vi "PmacProgParse.vi"(1 "Program Buffer String":string) -> (0 "Program VI State Cluster":T1={"Program Loaded"=FALSE, "Program Number i32"=1, "Coord Number i32"=1} {"Coord Number i32" min=1 max=8; "Program Number i32" min=1})   [LabVIEW 2020]
doc: "Parse Program Buffer to Program Number and Coord Number to run the program in. Provide the information in Program VI State Cluster. The program load state is not determined by this operation."
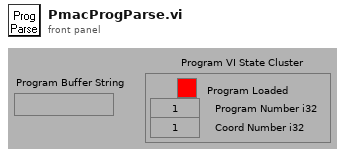
[diagram p1: front panel]
types:
  T1 = cluster{"Program Loaded":bool, "Program Number i32":i32, "Coord Number i32":i32}
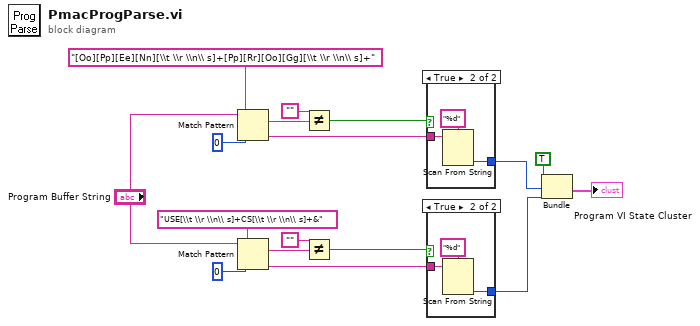
[diagram p0: block diagram]
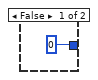
[diagram p2: hidden frame]
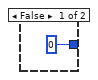
[diagram p3: hidden frame]
diagram:
  n1 = Match Pattern(string="Program Buffer String", regular expression="[Oo][Pp][Ee][Nn][\\t \\r \\n\\ s]+[Pp][Rr][Oo][Gg][\\t \\r \\n\\ s]+", offset (0)=0) -> (match substring=w9:string, after substring=w5:string)  [unwired: 2 out]
  n2 = Match Pattern(string="Program Buffer String", regular expression="USE[\\t \\r \\n\\ s]+CS[\\t \\r \\n\\ s]+&", offset (0)=0) -> (match substring=w8:string, after substring=w7:string)  [unwired: 2 out]
  n3 = Not Equal?(x="", y=w9) -> (x != y?=w6:bool)
  n4 = Not Equal?(x="", y=w8) -> (x != y?=w11:bool)
  n5 = case shown="True" w6 {
    tunnel: [0 w19] -> w3
    tunnel: w5 -> [_ w20]
    frame False {
    }
    frame True {
      n6 = Scan From String(format string="%d", input string=w20) -> (output 1=w19:i32)  [unwired: 2 in, 4 out]
    }
  }
  n7 = case shown="True" w11 {
    tunnel: [0 w23] -> w2
    tunnel: w7 -> [_ w24]
    frame False {
    }
    frame True {
      n8 = Scan From String(format string="%d", input string=w24) -> (output 1=w23:i32)  [unwired: 2 in, 4 out]
    }
  }
  n9 = Bundle(TRUE, w3, w2) -> (→"Program VI State Cluster":cluster{bool, i32, i32})  [unwired: 1 out]
